vi "Respond to Menu Event.vi"(8 "error in":errorcluster, 10 "Selection":string, 11 "Base Software in":refnum<class "Base Software.lvclass">) -> (0 "error out":errorcluster, 3 "Base Software out":refnum<class "Base Software.lvclass">)   [LabVIEW 2019, in "Base Software.lvlib" / "Main.lvlib" / "Base Software.lvclass"]
uses:
  Project/Base Software.lvclass
  C:/Users/Public/Documents/Development/builds/Engine/Engine.lvlibp/Project/Engine.lvclass
  builds/Engine/Engine.lvlibp/Custom Controls/System Status.ctl
  Project/Base Software.lvclass/Base Software.ctl
  Accessors/StateMachine/Write State.vi
  Accessors/StateMachine/Read State.vi
  Custom Controls/g_Identifiers.vi
  builds/Engine/Engine.lvlibp/Accessors/Read Self Q.vi
  GUI Support/State Machine Logic/Refresh State.vi
  Accessors/Buttons/Manual.vi
  <vilib>/ErrorRing/Error Ring.xnode
  builds/Engine/Actor Framework.lvlibp/1abvi3w/vi.lib/ActorFramework/Message Enqueuer/Message Enqueuer.lvclass
  builds/Engine/Actor Framework.lvlibp/1abvi3w/vi.lib/ActorFramework/Stop Msg/Stop Msg.lvclass
  builds/Engine/Engine.lvlibp/Project/Engine.lvclass
  builds/Engine/Engine.lvlibp/Engine Messages/Toggle Component Display Msg/Toggle Component Display Msg.lvclass
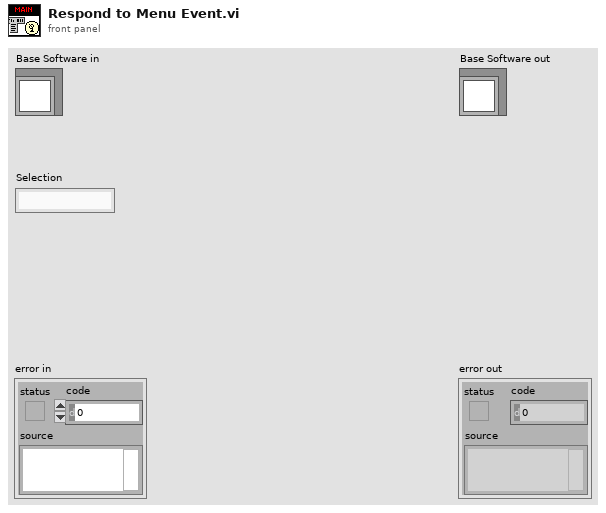
[diagram p1: front panel]
types:
  T1 = typedef "Engine.lvlibp/Engine.lvclass/System Status.ctl" = enum16{"Logged Off", "UUT_Info_Missing", "Idle", "Error", "Warning", "Loading", "Config", "Manual", "Automation", "Report_View", "Previous"}
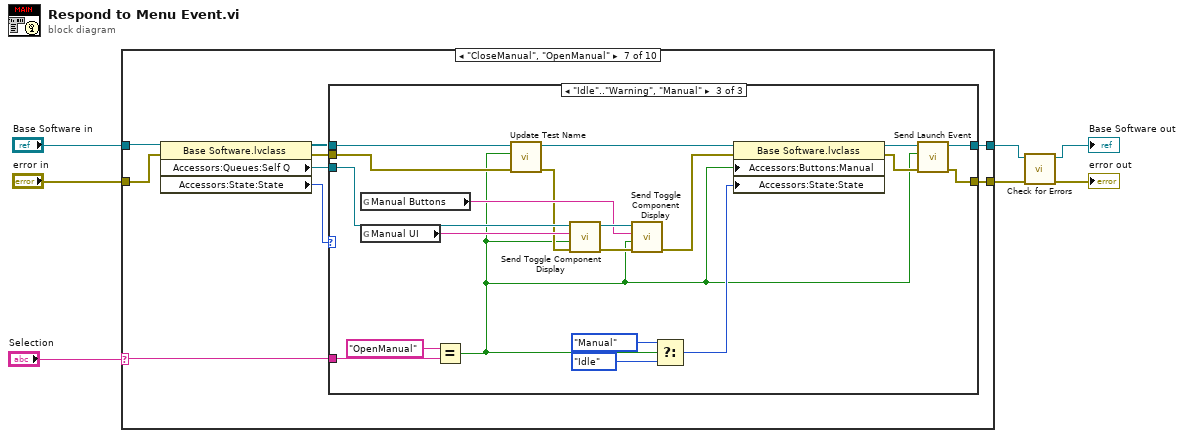
[diagram p0: block diagram]
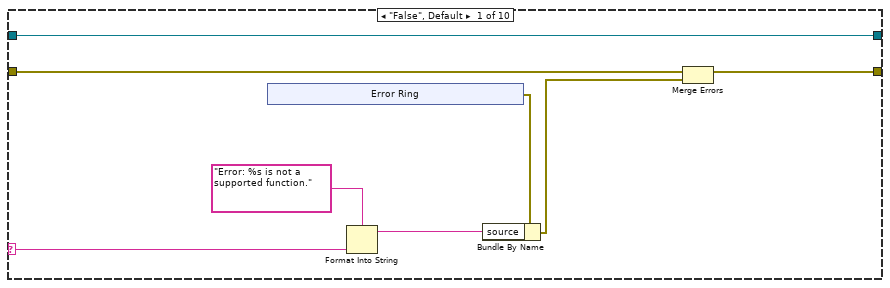
[diagram p2: hidden frame]
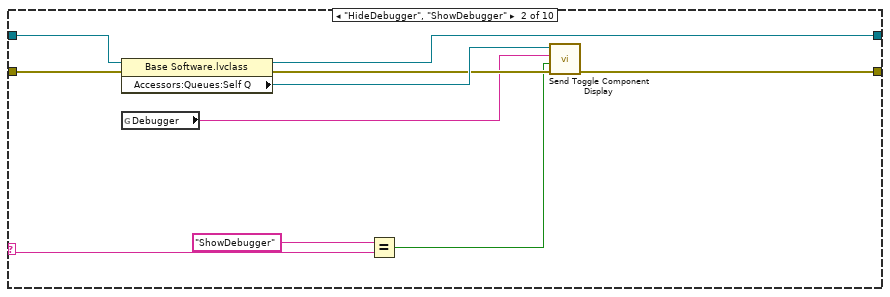
[diagram p3: hidden frame]
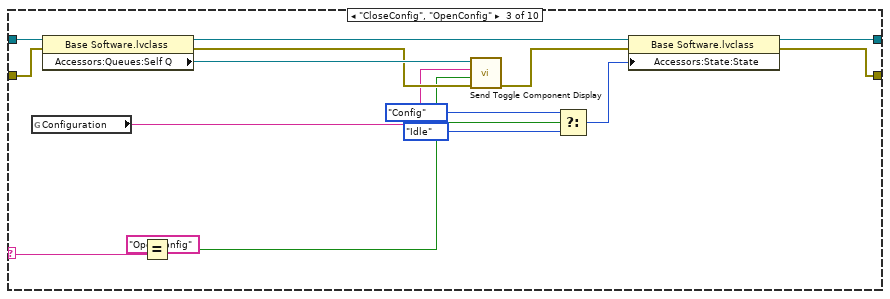
[diagram p4: hidden frame]
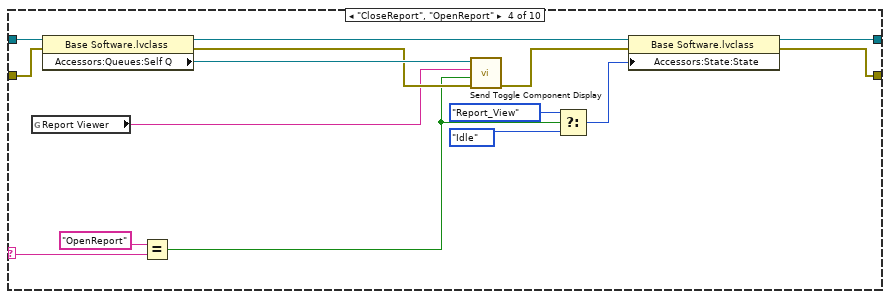
[diagram p5: hidden frame]
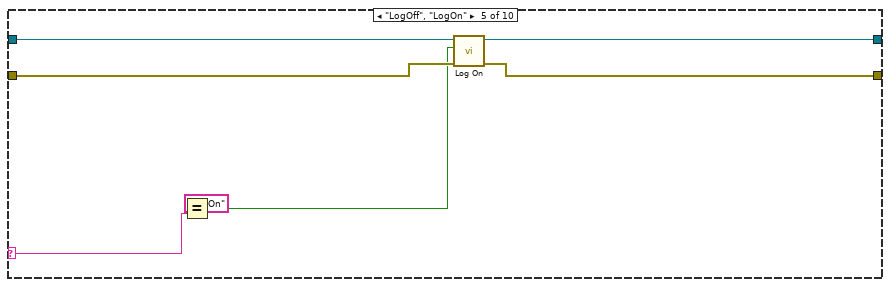
[diagram p6: hidden frame]
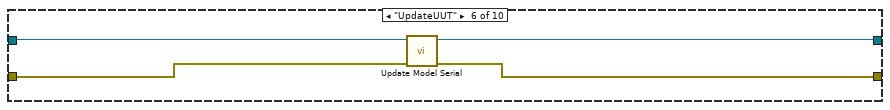
[diagram p7: hidden frame]
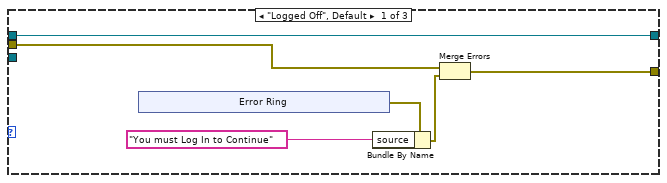
[diagram p8: hidden frame]
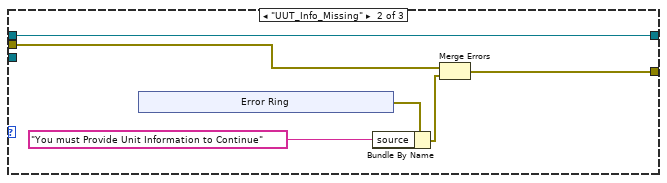
[diagram p9: hidden frame]
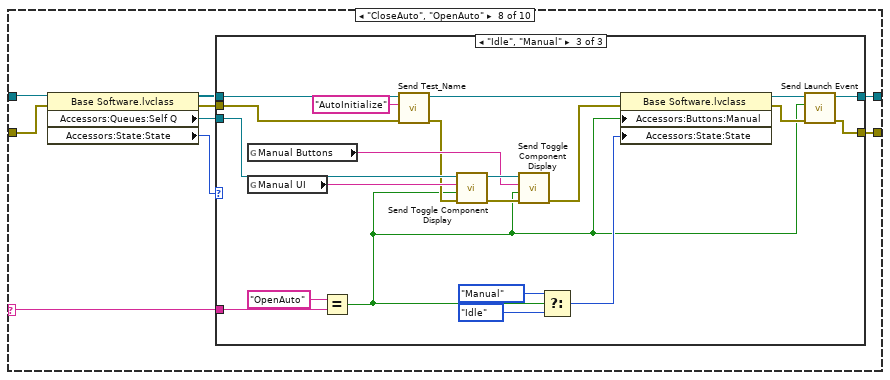
[diagram p10: hidden frame]
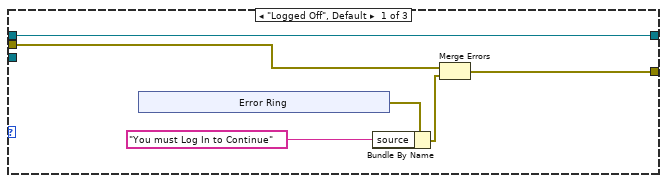
[diagram p11: hidden frame]
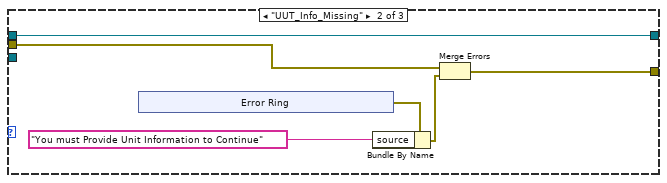
[diagram p12: hidden frame]
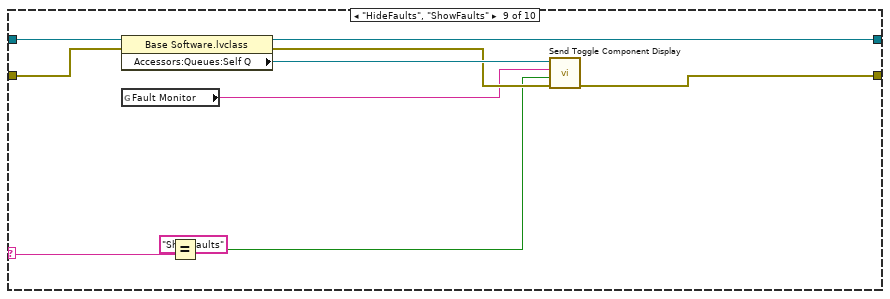
[diagram p13: hidden frame]
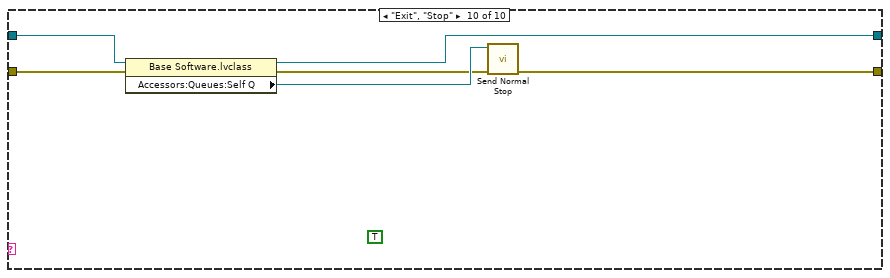
[diagram p14: hidden frame]
diagram:
  n1 = case shown="\"CloseManual\", \"OpenManual\"" "Selection" {
    selector: "Selection" -> [w9 w19 w36 w51 w58 _ w76 w119 w157 _]
    tunnel: "Base Software in" -> [w15 w26 w41 w56 w63 w67 w75 w118 w164 w169]
    tunnel: [w15 w24 w31 w46 w61 w64 w72 w115 w162 w168] -> w2
    tunnel: "error in" -> [w14 w25 w40 w55 w62 w66 w74 w117 w163 w170]
    tunnel: [w13 w21 w32 w47 w60 w65 w69 w112 w159 w165] -> w4
    frame "False", Default {
      n2 = xnode "Error Ring"() -> ("error out"=w12:errorcluster)
      n3 = Format Into String(format string="Error: %s is not a supported function.", w9) -> (resulting string=w8:string)  [unwired: 2 in, 1 out]
      n4 = Bundle By Name(cluster=w12, "source"=w8) -> (w11:errorcluster)
      n5 = Merge Errors(w14, w11) -> (w13:errorcluster)
    }
    frame "HideDebugger", "ShowDebugger" {
      n6 = property class="Base Software.lvclass"(reference=w26, error in=w25) -> (reference out=w24:refnum<class "Base Software.lvclass">, error out=w22:errorcluster, "Accessors:Queues:Self Q"=w23:refnum<class "Message Enqueuer.lvclass">)
      n7 = global read "g_Identifiers.vi" "Debugger"() -> (w20:string)
      n8 = Equal?(x="ShowDebugger", y=w19) -> (x = y?=w17:bool)
      n9 = call "Send Toggle Component Display.vi"("error in (no error)"=w22, "Show"=w17, "Identifier"=w20, "Message Enqueuer"=w23) -> ("error out"=w21:errorcluster)  [unwired: 6 in, 1 out]
    }
    frame "CloseConfig", "OpenConfig" {
      n10 = global read "g_Identifiers.vi" "Configuration"() -> (w37:string)
      n11 = property class="Base Software.lvclass"(reference=w41, error in=w40) -> (reference out=w34:refnum<class "Base Software.lvclass">, error out=w38:errorcluster, "Accessors:Queues:Self Q"=w39:refnum<class "Message Enqueuer.lvclass">)
      n12 = Equal?(x="OpenConfig", y=w36) -> (x = y?=w28:bool)
      n13 = call "Send Toggle Component Display.vi"("error in (no error)"=w38, "Show"=w28, "Identifier"=w37, "Message Enqueuer"=w39) -> ("error out"=w33:errorcluster)  [unwired: 6 in, 1 out]
      n14 = Select(t=System_Status."Config" ("Base:StateMachine:State"), s=w28, f=System_Status."Idle" ("Base:StateMachine:State")) -> (s? t:f=w27:T1)
      n15 = property class="Base Software.lvclass"(reference=w34, error in=w33, "Accessors:State:State"=w27) -> (reference out=w31:refnum<class "Base Software.lvclass">, error out=w32:errorcluster)
    }
    frame "CloseReport", "OpenReport" {
      n16 = global read "g_Identifiers.vi" "Report Viewer"() -> (w52:string)
      n17 = property class="Base Software.lvclass"(reference=w56, error in=w55) -> (reference out=w49:refnum<class "Base Software.lvclass">, error out=w53:errorcluster, "Accessors:Queues:Self Q"=w54:refnum<class "Message Enqueuer.lvclass">)
      n18 = Equal?(x="OpenReport", y=w51) -> (x = y?=w45:bool)
      n19 = call "Send Toggle Component Display.vi"("error in (no error)"=w53, "Show"=w45, "Identifier"=w52, "Message Enqueuer"=w54) -> ("error out"=w48:errorcluster)  [unwired: 6 in, 1 out]
      n20 = Select(t=System_Status."Report_View" ("Base:StateMachine:State"), s=w45, f=System_Status."Idle" ("Base:StateMachine:State")) -> (s? t:f=w42:T1)
      n21 = property class="Base Software.lvclass"(reference=w49, error in=w48, "Accessors:State:State"=w42) -> (reference out=w46:refnum<class "Base Software.lvclass">, error out=w47:errorcluster)
    }
    frame "LogOff", "LogOn" {
      n22 = Equal?(x="LogOn", y=w58) -> (x = y?=w57:bool)
      n23 = call "Log On.vi"("error in"=w62, "Log On"=w57, "Base Software in"=w63) -> ("error out"=w60:errorcluster, "Base Software out"=w61:refnum<class "Base Software.lvclass">)  [unwired: 7 in]
    }
    frame "UpdateUUT" {
      n24 = call "Update Model Serial.vi"("error in"=w66, "Base Software in"=w67) -> ("error out"=w65:errorcluster, "Base Software out"=w64:refnum<class "Base Software.lvclass">)  [unwired: 7 in, 1 out]
    }
    frame "CloseManual", "OpenManual" {
      n25 = property class="Base Software.lvclass"(reference=w75, error in=w74) -> (reference out=w73:refnum<class "Base Software.lvclass">, error out=w70:errorcluster, "Accessors:Queues:Self Q"=w71:refnum<class "Message Enqueuer.lvclass">, "Accessors:State:State"=w68:T1)
      n26 = case shown="\"Idle\"..\"Warning\", \"Manual\"" w68 {
        tunnel: w76 -> [_ _ w110]
        tunnel: w73 -> [w82 w89 w95]
        tunnel: [w82 w89 w97] -> w72
        tunnel: w71 -> [_ _ w108]
        tunnel: w70 -> [w81 w88 w94]
        tunnel: [w80 w87 w96] -> w69
        frame "Logged Off", Default {
          n27 = xnode "Error Ring"() -> ("error out"=w79:errorcluster)
          n28 = Bundle By Name(cluster=w79, "source"="You must Log In to Continue") -> (w78:errorcluster)
          n29 = Merge Errors(w81, w78) -> (w80:errorcluster)
        }
        frame "UUT_Info_Missing" {
          n30 = xnode "Error Ring"() -> ("error out"=w86:errorcluster)
          n31 = Bundle By Name(cluster=w86, "source"="You must Provide Unit Information to Continue") -> (w85:errorcluster)
          n32 = Merge Errors(w88, w85) -> (w87:errorcluster)
        }
        frame "Idle".."Warning", "Manual" {
          n33 = global read "g_Identifiers.vi" "Manual Buttons"() -> (w101:string)
          n34 = global read "g_Identifiers.vi" "Manual UI"() -> (w107:string)
          n35 = Equal?(x="OpenManual", y=w110) -> (x = y?=w91:bool)
          n36 = call "Update Test Name.vi"("error in"=w94, "Show"=w91, "Base Software in"=w95) -> ("error out"=w93:errorcluster, "Base Software out"=w92:refnum<class "Base Software.lvclass">)  [unwired: 7 in]
          n37 = call "Send Toggle Component Display.vi"("error in (no error)"=w93, "Show"=w91, "Identifier"=w107, "Message Enqueuer"=w108) -> ("error out"=w104:errorcluster, "Message Enqueuer out"=w103:refnum<class "Message Enqueuer.lvclass">)  [unwired: 6 in]
          n38 = call "Send Toggle Component Display.vi"("error in (no error)"=w104, "Show"=w91, "Identifier"=w101, "Message Enqueuer"=w103) -> ("error out"=w102:errorcluster)  [unwired: 6 in, 1 out]
          n39 = Select(t=System_Status."Manual" ("Base:StateMachine:State"), s=w91, f=System_Status."Idle" ("Base:StateMachine:State")) -> (s? t:f=w100:T1)
          n40 = property class="Base Software.lvclass"(reference=w92, error in=w102, "Accessors:Buttons:Manual"=w91, "Accessors:State:State"=w100) -> (reference out=w99:refnum<class "Base Software.lvclass">, error out=w98:errorcluster)
          n41 = call "Send Launch Event.vi"("error in"=w98, "Launch"=w91, "Engine in"=w99) -> ("error out"=w96:errorcluster, "Engine out"=w97:refnum<class "Base Software.lvclass">)  [unwired: 7 in]
        }
      }
    }
    frame "CloseAuto", "OpenAuto" {
      n42 = property class="Base Software.lvclass"(reference=w118, error in=w117) -> (reference out=w116:refnum<class "Base Software.lvclass">, error out=w113:errorcluster, "Accessors:Queues:Self Q"=w114:refnum<class "Message Enqueuer.lvclass">, "Accessors:State:State"=w111:T1)
      n43 = case shown="\"Idle\", \"Manual\"" w111 {
        tunnel: w119 -> [_ _ w154]
        tunnel: w116 -> [w125 w132 w139]
        tunnel: [w125 w132 w141] -> w115
        tunnel: w114 -> [_ _ w152]
        tunnel: w113 -> [w124 w131 w137]
        tunnel: [w123 w130 w140] -> w112
        frame "Logged Off", Default {
          n44 = xnode "Error Ring"() -> ("error out"=w122:errorcluster)
          n45 = Bundle By Name(cluster=w122, "source"="You must Log In to Continue") -> (w121:errorcluster)
          n46 = Merge Errors(w124, w121) -> (w123:errorcluster)
        }
        frame "UUT_Info_Missing" {
          n47 = xnode "Error Ring"() -> ("error out"=w129:errorcluster)
          n48 = Bundle By Name(cluster=w129, "source"="You must Provide Unit Information to Continue") -> (w128:errorcluster)
          n49 = Merge Errors(w131, w128) -> (w130:errorcluster)
        }
        frame "Idle", "Manual" {
          n50 = global read "g_Identifiers.vi" "Manual Buttons"() -> (w145:string)
          n51 = global read "g_Identifiers.vi" "Manual UI"() -> (w151:string)
          n52 = Equal?(x="OpenAuto", y=w154) -> (x = y?=w135:bool)
          n53 = call "Send Test_Name.vi"("error in"=w137, "Test Name"="AutoInitialize", "Engine in"=w139) -> ("error out"=w136:errorcluster, "Engine out"=w138:refnum<class "Base Software.lvclass">)  [unwired: 7 in]
          n54 = call "Send Toggle Component Display.vi"("error in (no error)"=w136, "Show"=w135, "Identifier"=w151, "Message Enqueuer"=w152) -> ("error out"=w148:errorcluster, "Message Enqueuer out"=w147:refnum<class "Message Enqueuer.lvclass">)  [unwired: 6 in]
          n55 = call "Send Toggle Component Display.vi"("error in (no error)"=w148, "Show"=w135, "Identifier"=w145, "Message Enqueuer"=w147) -> ("error out"=w146:errorcluster)  [unwired: 6 in, 1 out]
          n56 = Select(t=System_Status."Manual" ("Base:StateMachine:State"), s=w135, f=System_Status."Idle" ("Base:StateMachine:State")) -> (s? t:f=w144:T1)
          n57 = property class="Base Software.lvclass"(reference=w138, error in=w146, "Accessors:Buttons:Manual"=w135, "Accessors:State:State"=w144) -> (reference out=w143:refnum<class "Base Software.lvclass">, error out=w142:errorcluster)
          n58 = call "Send Launch Event.vi"("error in"=w142, "Launch"=w135, "Engine in"=w143) -> ("error out"=w140:errorcluster, "Engine out"=w141:refnum<class "Base Software.lvclass">)  [unwired: 7 in]
        }
      }
    }
    frame "HideFaults", "ShowFaults" {
      n59 = property class="Base Software.lvclass"(reference=w164, error in=w163) -> (reference out=w162:refnum<class "Base Software.lvclass">, error out=w160:errorcluster, "Accessors:Queues:Self Q"=w161:refnum<class "Message Enqueuer.lvclass">)
      n60 = global read "g_Identifiers.vi" "Fault Monitor"() -> (w158:string)
      n61 = Equal?(x="ShowFaults", y=w157) -> (x = y?=w155:bool)
      n62 = call "Send Toggle Component Display.vi"("error in (no error)"=w160, "Show"=w155, "Identifier"=w158, "Message Enqueuer"=w161) -> ("error out"=w159:errorcluster)  [unwired: 6 in, 1 out]
    }
    frame "Exit", "Stop" {
      (unwired) TRUE
      n63 = property class="Base Software.lvclass"(reference=w169, error in=w170) -> (reference out=w168:refnum<class "Base Software.lvclass">, error out=w166:errorcluster, "Accessors:Queues:Self Q"=w167:refnum<class "Message Enqueuer.lvclass">)
      n64 = call "Send Normal Stop.vi"("error in (no error)"=w166, "Message Enqueuer"=w167) -> ("error out"=w165:errorcluster)  [unwired: 9 in]
    }
  }
  n65 = call "Check for Errors.vi"("error in"=w4, "Engine in"=w2) -> ("error out"=→"error out":errorcluster, "Engine out"=→"Base Software out":refnum<class "Base Software.lvclass">)  [unwired: 8 in]
